vi "UDMA_READ_FIFO_CONT.vi"(0 "TCP Network Connection in":refnum<k5>, 5 "error in (no error)":errorcluster) -> (14 "TCP Network Connection out":refnum<k5>, 16 "Oscilloscope":u32[](graph), 18 "Status":u8[](array[numeric]), 19 "error out":errorcluster)   [LabVIEW 2019]
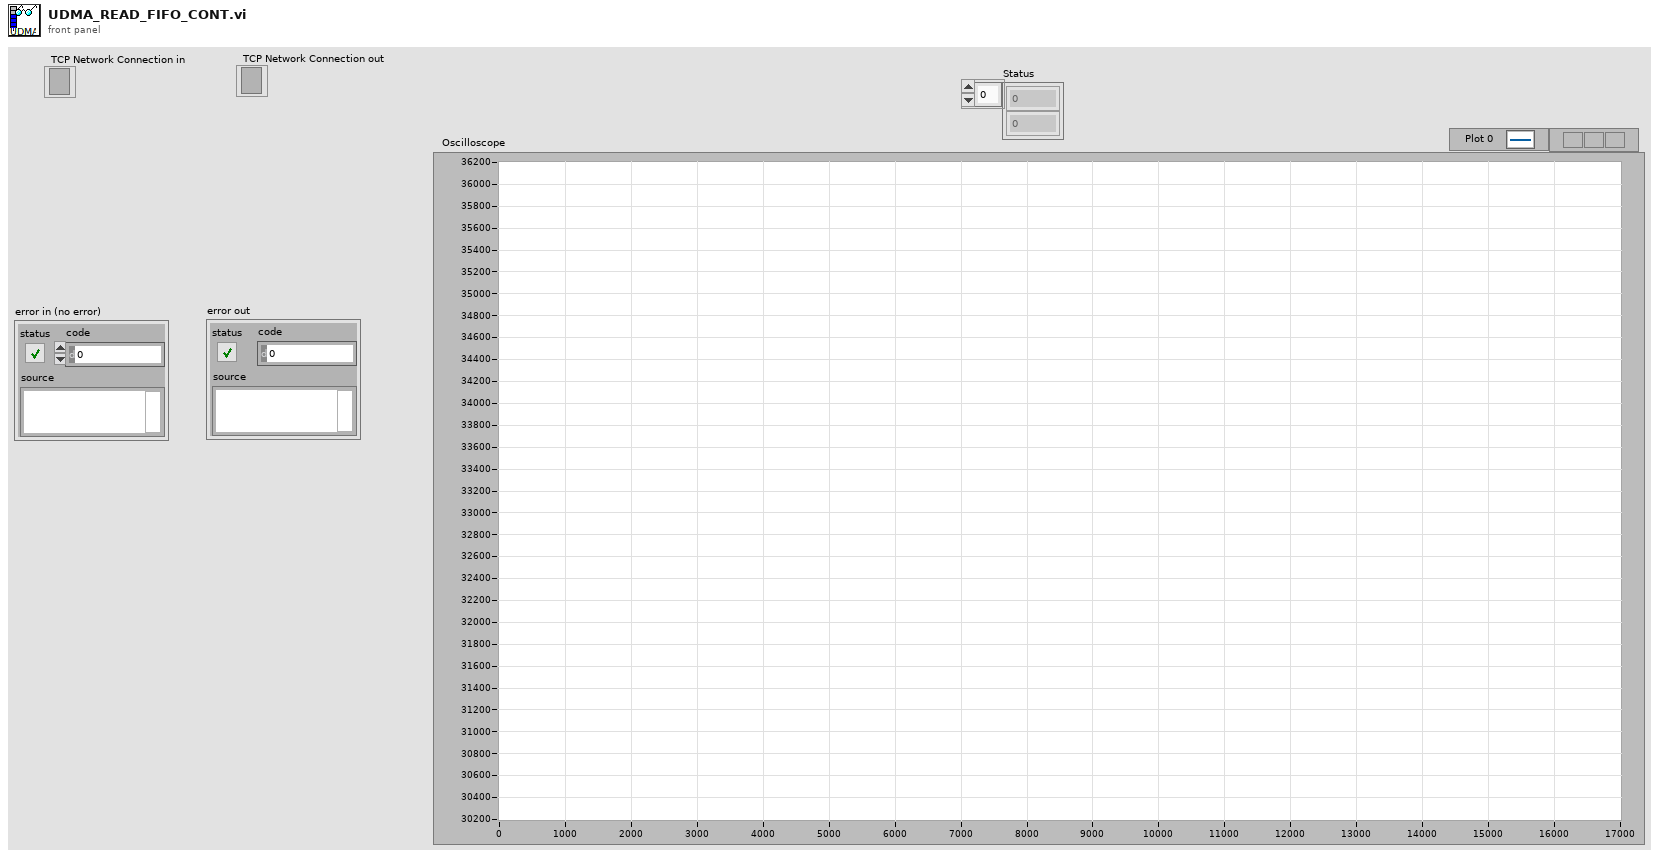
[diagram p1: front panel]
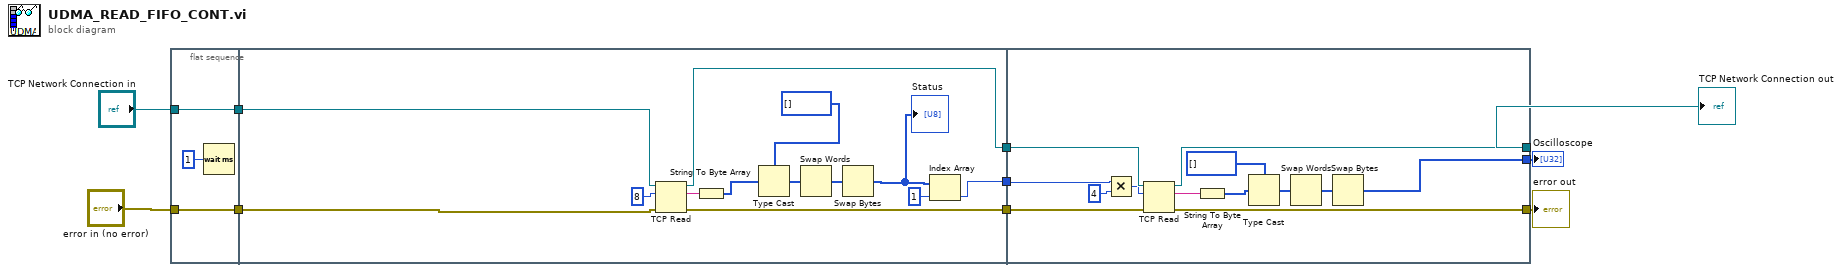
[diagram p0: block diagram]
diagram:
  n1 = flat-sequence {
    tunnel: "TCP Network Connection in" -> [w12]
    tunnel: "error in (no error)" -> [w13]
    tunnel: [w13] -> w2
    tunnel: [w12] -> w1
    tunnel: [w26] -> w5
    tunnel: [w17] -> w4
    tunnel: [w25] -> w3
    tunnel: w2 -> [w14]
    tunnel: w1 -> [w15]
    tunnel: [w37] -> w6
    tunnel: [w38] -> w8
    tunnel: [w39] -> w7
    tunnel: w3 -> [w36]
    tunnel: w4 -> [w27]
    tunnel: w5 -> [w35]
    frame #0 {
      n2 = Wait (ms)(milliseconds to wait=u32 1) -> ()  [unwired: 1 out]
    }
    frame #1 {
      n3 = TCP Read(connection ID=w15, bytes to read=8, error in (no error)=w14) -> (connection ID out=w25:refnum<k5>, data out=w24:string, error out=w26:errorcluster)  [unwired: 2 in]
      n4 = String To Byte Array(string=w24) -> (unsigned byte array=w22:u8[])
      n5 = Type Cast(type=u32[] [], x=w22) -> (*(type *) &x=w21:u32[])
      n6 = Swap Words(1:w21) -> (0:w20:u32[])
      n7 = Swap Bytes(anything=w20) -> (byte swapped=w16:u32[])
      "Status" <- w16
      n8 = Index Array(array=w16, index=1) -> (element=w17:u32)
    }
    frame #2 {
      n9 = Multiply(x=w27, y=u32 4) -> (x*y=w34:u32)
      n10 = TCP Read(connection ID=w36, bytes to read=w34, error in (no error)=w35) -> (connection ID out=w39:refnum<k5>, data out=w28:string, error out=w38:errorcluster)  [unwired: 2 in]
      n11 = String To Byte Array(string=w28) -> (unsigned byte array=w32:u8[])
      n12 = Type Cast(type=u32[] [], x=w32) -> (*(type *) &x=w30:u32[])
      n13 = Swap Words(1:w30) -> (0:w29:u32[])
      n14 = Swap Bytes(anything=w29) -> (byte swapped=w37:u32[])
    }
  }
  "error out" <- w8
  "TCP Network Connection out" <- w7
  "Oscilloscope" <- w6
